vi "c2f(SubVI).vi"(1 "Degrees C":dbl, 2 "Boolean":bool) -> (0 "Numeric":dbl)   [LabVIEW 2015]
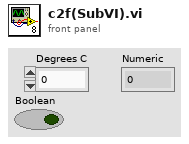
[diagram p1: front panel]
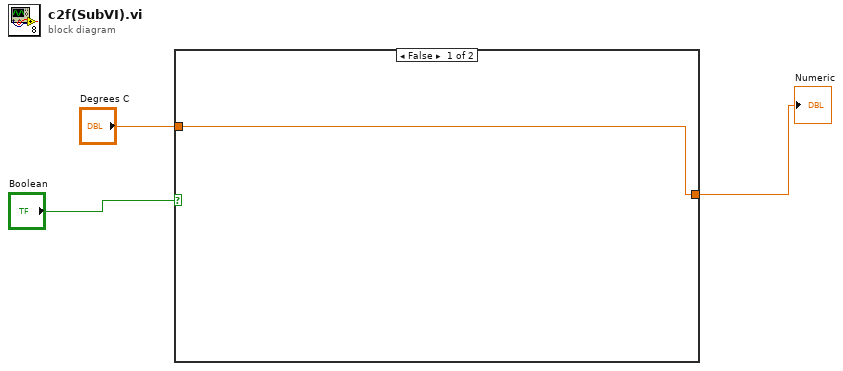
[diagram p0: block diagram]
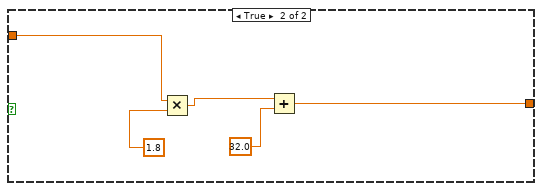
[diagram p2: hidden frame]
diagram:
  n1 = case shown="False" "Boolean" {
    tunnel: "Degrees C" -> [w4 w6]
    tunnel: [w4 w5] -> w2
    frame False {
    }
    frame True {
      n2 = Multiply(x=w6, y=1.8) -> (x*y=w8:dbl)
      n3 = Add(x=w8, y=32.0) -> (x+y=w5:dbl)
    }
  }
  "Numeric" <- w2
